vi "Read Grouped Tags.vi"(8 "error in (no error)":errorcluster, 11 "Group":string) -> (0 "error out":errorcluster, 2 "Data":T1)   [LabVIEW 2010, in "Current Value Table.lvlib"]
doc: "This VI will read an entire group as defined during tag creation or by the FormGroup VI. This VI functions as both the normal and static versions of the group read, as the small performance drop from the group name check is insignificant for reasonably sized groups."
uses:
  Current Value Table.lvlib
  Type Defs/Group Data.ctl
  FGVs/Group Memory Methods.ctl
  Read Index Set.vi
  DataTypes/Double_Read Index Set.vi
  DataTypes/Array of String_Read Index Set.vi
  DataTypes/Array of Boolean_Read Index Set.vi
  DataTypes/Array of Single_Read Index Set.vi
  DataTypes/Array of Double_Read Index Set.vi
  DataTypes/Array of I8_Read Index Set.vi
  DataTypes/Array of I16_Read Index Set.vi
  DataTypes/Array of I32_Read Index Set.vi
  DataTypes/Array of I64_Read Index Set.vi
  DataTypes/Array of U64_Read Index Set.vi
  DataTypes/Array of U32_Read Index Set.vi
  DataTypes/Array of U16_Read Index Set.vi
  DataTypes/Array of U8_Read Index Set.vi
  DataTypes/Boolean_Read Index Set.vi
  DataTypes/String_Read Index Set.vi
  DataTypes/U8_Read Index Set.vi
  DataTypes/U16_Read Index Set.vi
  DataTypes/U32_Read Index Set.vi
  DataTypes/U64_Read Index Set.vi
  DataTypes/I8_Read Index Set.vi
  DataTypes/I16_Read Index Set.vi
  DataTypes/I32_Read Index Set.vi
  DataTypes/I64_Read Index Set.vi
  DataTypes/Single_Read Index Set.vi
  Memory Block.vi
  DataTypes/Double_Memory Block.vi
  DataTypes/Array of String_Memory Block.vi
  DataTypes/Array of Boolean_Memory Block.vi
  DataTypes/Array of Single_Memory Block.vi
  DataTypes/Array of Double_Memory Block.vi
  DataTypes/Array of I8_Memory Block.vi
  DataTypes/Array of I16_Memory Block.vi
  DataTypes/Array of I32_Memory Block.vi
  DataTypes/Array of I64_Memory Block.vi
  DataTypes/Array of U64_Memory Block.vi
  DataTypes/Array of U32_Memory Block.vi
  DataTypes/Array of U16_Memory Block.vi
  DataTypes/Array of U8_Memory Block.vi
  DataTypes/Boolean_Memory Block.vi
  DataTypes/String_Memory Block.vi
  DataTypes/U8_Memory Block.vi
  DataTypes/U16_Memory Block.vi
  DataTypes/U32_Memory Block.vi
  DataTypes/U64_Memory Block.vi
  DataTypes/I8_Memory Block.vi
  DataTypes/I16_Memory Block.vi
  DataTypes/I32_Memory Block.vi
  DataTypes/I64_Memory Block.vi
  DataTypes/Single_Memory Block.vi
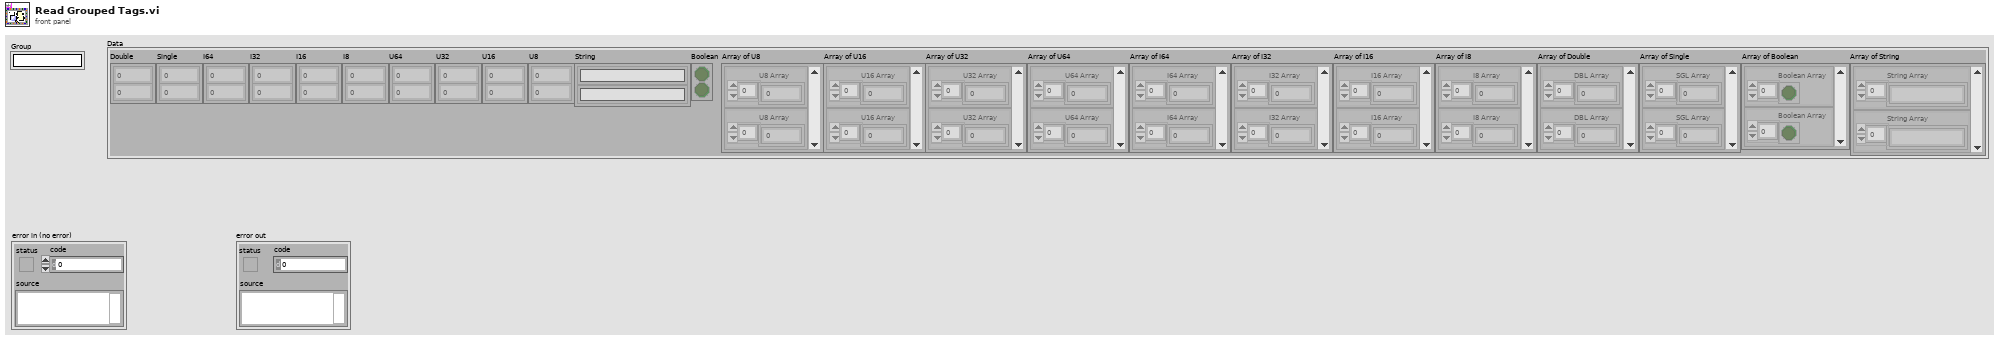
[diagram p1: front panel]
types:
  T1 = typedef "Current Value Table.lvlib/Group Data.ctl" = cluster{"Double":dbl[], "Single":sgl[], "I64":i64[], "I32":i32[], "I16":i16[], "I8":i8[], "U64":u64[], "U32":u32[], "U16":u16[], "U8":u8[], "String":string[], "Boolean":bool[], "Array of U8":cluster{"U8 Array":u8[]}[], "Array of U16":cluster{"U16 Array":u16[]}[], "Array of U32":cluster{"U32 Array":u32[]}[], "Array of U64":cluster{"U64 Array":u64[]}[], "Array of I64":cluster{"I64 Array":i64[]}[], "Array of I32":cluster{"I32 Array":i32[]}[], "Array of I16":cluster{"I16 Array":i16[]}[], "Array of I8":cluster{"I8 Array":i8[]}[], "Array of Double":cluster{"DBL Array":dbl[]}[], "Array of Single":cluster{"SGL Array":sgl[]}[], "Array of Boolean":cluster{"Boolean Array":bool[]}[], "Array of String":cluster{"String Array":string[]}[]}
  T2 = typedef "Current Value Table.lvlib/Typed Index Set.ctl" = cluster{"Data Type":T3, "Indices":i32[]}
  T3 = typedef "Current Value Table.lvlib/Data Types.ctl" = enum16{"Double", "Single", "I64", "I32", "I16", "I8", "U64", "U32", "U16", "U8", "String", "Boolean", "Array of U8", "Array of U16", "Array of U32", "Array of U64", "Array of I64", "Array of I32", "Array of I16", "Array of I8", "Array of Double", "Array of Single", "Array of Boolean", "Array of String"}
  T4 = typedef "Current Value Table.lvlib/Group Memory Methods.ctl" = enum16{"Clear", "Read Indices in Group", "List Groups", "List Tags by Type", "List Tags", "Delete Group", "Check Group Existence", "Create Group"}
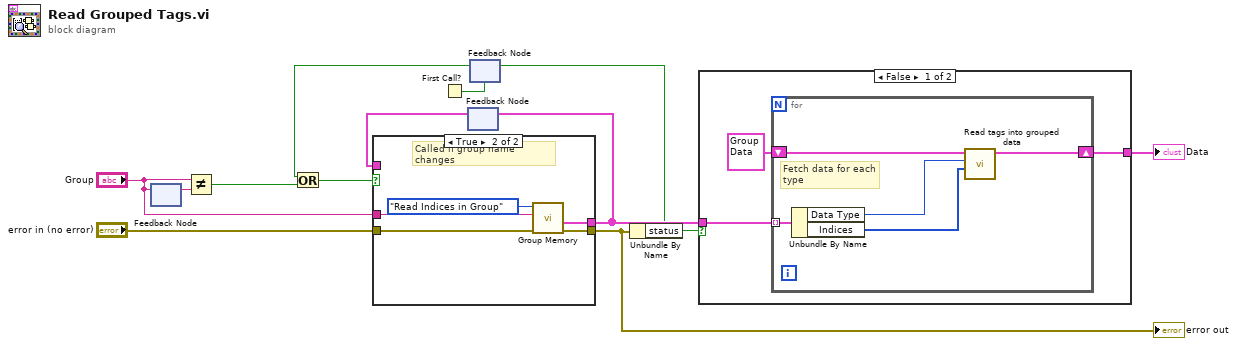
[diagram p0: block diagram]
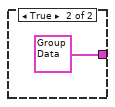
[diagram p2: hidden frame]
diagram:
  n1 = feedback #1() -> (w11:string)  [unwired: 1 in]
  n2 = feedback-in #1("Group") -> ()
  n3 = Not Equal?(x="Group", y=w11) -> (x != y?=w4:bool)
  n4 = First Call?() -> (First Call?: T/F=w5:bool)
  n5 = feedback #2() -> (w8:T2[])  [unwired: 1 in]
  n6 = feedback #3(w5) -> (w2:bool)
  n7 = Or(x=w2, y=w4) -> (x .or. y?=w3:bool)
  n8 = case shown="True" w3 {
    tunnel: [w14 w19] -> w6
    tunnel: "error in (no error)" -> [w14 w17]
    tunnel: "Group" -> [_ w16]
    tunnel: [w13 w18] -> w9
    tunnel: w8 -> [w13 _]
    frame False {
      # "Buffer lookup data"
    }
    frame True {
      # "Called if group name changes"
      n9 = call "Group Memory.vi"("error in (no error)"=w17, "Group"=w16, "Method"=Group_Memory_Methods."Read Indices in Group") -> ("error out"=w19:errorcluster, "Group Indices Out"=w18:T2[])  [unwired: 5 in, 2 out]
    }
  }
  "error out" <- w6
  n10 = feedback-in #2(w9) -> ()
  n11 = Unbundle By Name(w6) -> ("status"=w1:bool)
  n12 = feedback-in #3(w1) -> ()
  n13 = case shown="False" w1 {
    tunnel: w9 -> [w22 _]
    tunnel: [w20 T1 {"Double"=[], "Single"=[], "I64"=[], "I32"=[], "I16"=[], "I8"=[], "U64"=[], "U32"=[], "U16"=[], "U8"=[], "String"=[], "Boolean"=[], "Array of U8"=[], "Array of U16"=[], "Array of U32"=[], "Array of U64"=[], "Array of I64"=[], "Array of I32"=[], "Array of I16"=[], "Array of I8"=[], "Array of Double"=[], "Array of Single"=[], "Array of Boolean"=[], "Array of String"=[]} ("Data")] -> w7
    frame False {
      n14 = for {
        tunnel: w22 -> [w27] mode=indexing
        shift-right: [w23] -> w20
        shift-left: T1 {"Double"=[], "Single"=[], "I64"=[], "I32"=[], "I16"=[], "I8"=[], "U64"=[], "U32"=[], "U16"=[], "U8"=[], "String"=[], "Boolean"=[], "Array of U8"=[], "Array of U16"=[], "Array of U32"=[], "Array of U64"=[], "Array of I64"=[], "Array of I32"=[], "Array of I16"=[], "Array of I8"=[], "Array of Double"=[], "Array of Single"=[], "Array of Boolean"=[], "Array of String"=[]} ("Data") -> [w24]
        # "Fetch data for each\ntype"
        n15 = Unbundle By Name(w27) -> ("Data Type"=w26:T3, "Indices"=w25:i32[])
        n16 = call "Read tags into grouped data.vi"("Indices"=w25, "Data Type"=w26, "Data in"=w24) -> ("Data out"=w23:T1)  [unwired: 8 in]
      }
    }
    frame True {
    }
  }
  "Data" <- w7
